vi "ScopeSettingsToH5.vi"(8 "error in (no error)":errorcluster, 10 "Cluster":T2, 11 "Refnum in":T1) -> (0 "error out":errorcluster, 1 "HDF5 Group Ref":T1, 3 "Refnum out":T1)   [LabVIEW 2011]
uses:
  <vilib>/UPVI/lvhdf5/library.llb/HDF5 Ref.ctl
  <vilib>/UPVI/lvhdf5/attribute.llb/LVH5A Operation.ctl
  <vilib>/Utility/miscctls.llb/LVRectTypeDef.ctl
  <vilib>/UPVI/lvhdf5/dataset.llb/LVH5D Operation.ctl
  <vilib>/UPVI/lvhdf5/group.llb/H5G_obj_t.ctl
  <vilib>/UPVI/lvhdf5/identifier.llb/Not an HDF5 Refnum Constant.vi
  <vilib>/UPVI/lvhdf5/common.llb/To HDF5 Ref.vi
  <vilib>/UPVI/lvhdf5/group.llb/OpenCreateGroup (String).vi
  <vilib>/UPVI/lvhdf5/attribute.llb/Write Multiple Attributes.vi
  <vilib>/Utility/VariantDataType/GetClusterInfo.vi
  <vilib>/Utility/VariantDataType/GetTypeInfo.vi
  <vilib>/UPVI/lvhdf5/utility.llb/Select HDF5 Dialog.vi
  <vilib>/UPVI/lvhdf5/utility.llb/Select HDF5 Dialog (Object Only).vi
  <vilib>/UPVI/lvhdf5/dataset.llb/Simple H5Dwrite (Variant).vi
  <vilib>/UPVI/lvhdf5/dataset.llb/H5Dclose.vi
  <vilib>/UPVI/lvhdf5/dataset.llb/Write Dataset with Attributes.xnode
  <vilib>/UPVI/lvhdf5/attribute.llb/Cluster to Attribute Array.xnode
  <vilib>/UPVI/lvhdf5/file.llb/H5Fclose.vi
  <vilib>/Utility/error.llb/Error Cluster From Error Code.vi
  <vilib>/UPVI/lvhdf5/dataset.llb/OpenCreateReplace Dataset by Element Type.vi
  <vilib>/UPVI/lvhdf5/dataspace.llb/H5Sselect_hyperslab.vi
  <vilib>/UPVI/lvhdf5/dataset.llb/H5Dwrite (Variant).vi
  <vilib>/UPVI/lvhdf5/dataset.llb/H5Dget_space.vi
  <vilib>/UPVI/lvhdf5/attribute.llb/private/LVH5AwriteWDTAttrs.vi
  <vilib>/UPVI/lvhdf5/dataspace.llb/H5Sclose.vi
  <vilib>/UPVI/lvhdf5/file.llb/OpenCreateReplace HDF5 File.vi
  <vilib>/UPVI/lvhdf5/file.llb/LVH5F Operation.ctl
  <vilib>/UPVI/lvhdf5/utility.llb/Select HDF5 Dialog (File and Object).vi
  <vilib>/Utility/VariantDataType/VariantType.lvlib
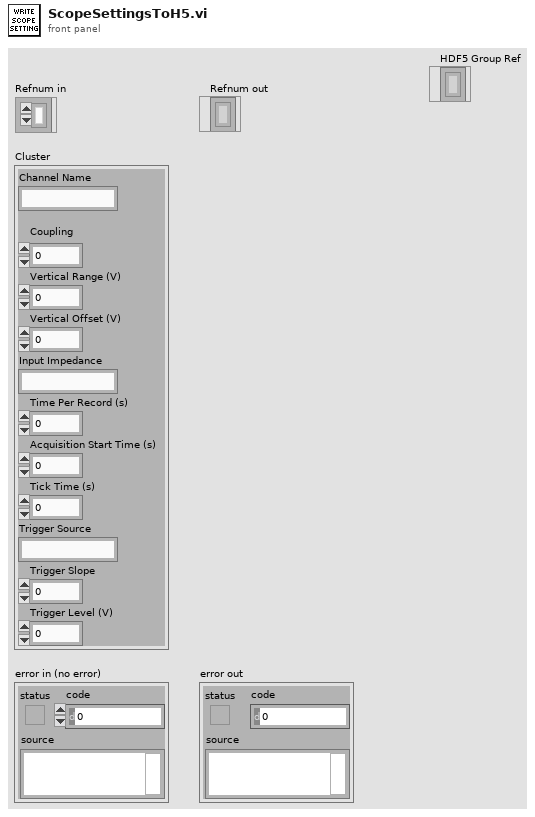
[diagram p1: front panel]
types:
  T1 = typedef "HDF5 Ref.ctl" = refnum<k1>
  T2 = cluster{"Channel Name":string, "\nCoupling":i32, "Vertical Range (V)":dbl, "Vertical Offset (V)":dbl, "Input Impedance":string, "Time Per Record (s)":dbl, "Acquisition Start Time (s)":dbl, "Tick Time (s)":dbl, "Trigger Source":string, "Trigger Slope":i32, "Trigger Level (V)":dbl}
  T3 = cluster{"Scope Model":string, "Trigger Coupling info":string, "Trigger Slope info":string}
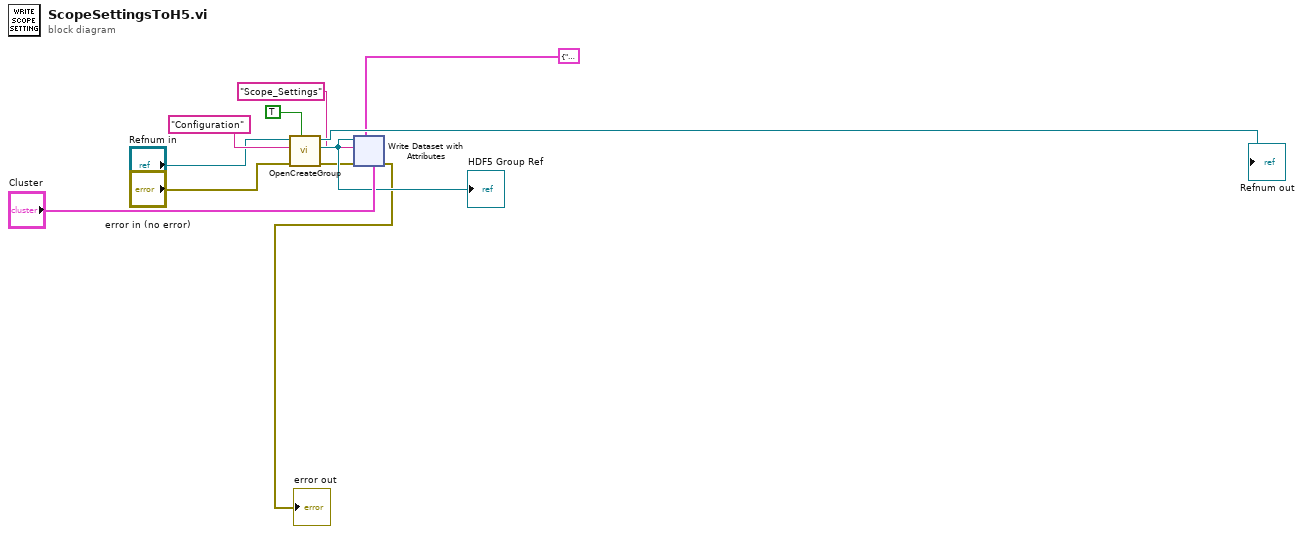
[diagram p0: block diagram]
diagram:
  n1 = call-poly <vilib>:"OpenCreateGroup.vi"("Create if not found (F)"=TRUE, "error in (no error)"="error in (no error)", "Group"="Configuration", "HDF5 Ref"="Refnum in") -> ("error out"=w6:errorcluster, "HDF5 Group Ref"=w8:T1, "HDF5 Ref out"=→"Refnum out":T1)  [unwired: 5 in]
  "HDF5 Group Ref" <- w8
  n2 = xnode "Write Dataset with Attributes"("Dataset Path"="Scope_Settings", "error in (no error)"=w6, "HDF5 Path or Ref"=w8, "Attribute Value(s)"=T3 {"Scope Model"="TDS3054", "Trigger Coupling info"="0 = AC, 1 = DC, 2 = GND", "Trigger Slope info"="0 = Positive, 1 = Negative"}, "Data"="Cluster") -> ("error out"=→"error out":errorcluster)  [unwired: 3 in, 2 out]
